vi "ChirpSourceGen(SubVI).vi"(3 "Frequency2(Hz)":dbl=30000.0 format="%#_6p", 4 "Frequency1(Hz)":dbl=30000.0 format="%#_6p", 5 "Pulse length(sec)":dbl=30000.0 format="%#_6p", 6 "Fs(Hz)":dbl=30000.0 format="%#_6p") -> (0 "dt":dbl, 1 "Chirp(F2-1)":dbl[](array[numeric]), 2 "Chirp(F1-2)":dbl[](array[numeric]))   [LabVIEW 2017]
uses:
  <vilib>/Analysis/NI_AALBase.lvlib
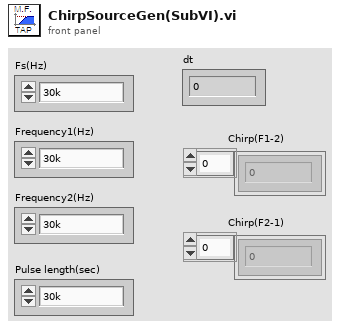
[diagram p1: front panel]
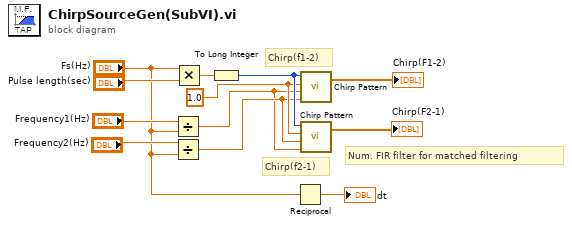
[diagram p0: block diagram]
diagram:
  w7 = 1.0 ("amplitude")
  # "Num. FIR filter for matched filtering"
  # "Chirp(f2-1)"
  # "Chirp(f1-2)"
  n1 = Divide(x="Frequency1(Hz)", y="Fs(Hz)") -> (x/y=w5:dbl)
  n2 = Divide(x="Frequency2(Hz)", y="Fs(Hz)") -> (x/y=w6:dbl)
  n3 = Multiply(x="Fs(Hz)", y="Pulse length(sec)") -> (x*y=w11:dbl)
  n4 = To Long Integer(number=w11) -> (32bit integer=w8:i32)
  n5 = Reciprocal(x="Fs(Hz)") -> (1/x=→"dt":dbl)
  n6 = call <vilib>:"Chirp Pattern.vi"("f2"=w6, "f1"=w5, "amplitude"=w7, "samples"=w8) -> ("Chirp Pattern"=→"Chirp(F1-2)":dbl[])  [unwired: 1 out]
  n7 = call <vilib>:"Chirp Pattern.vi"("f2"=w5, "f1"=w6, "amplitude"=w7, "samples"=w8) -> ("Chirp Pattern"=→"Chirp(F2-1)":dbl[])  [unwired: 1 out]
